vi "Compute DistanceTo AprilTag Ver 2.vi"(8 "Height to center of target from floor (hp (in))":dbl=10.875 format="%#_13g", 9 "Screen resolution pixels Height (Ry)":dbl=600.0 format="%#_13g", 10 "Target Vertical pixels bottom - top (pixels)":dbl=-46.076202392578125 format="%#_13g", 11 "Robot Calibration Cluster":T1={"Camera Height on robot (in)"=6.0, "Camera Angle on the robot (deg)"=5.0, "Camera FOV Vert View Angle (deg)"=1.0, "Camera FOV Hor View Angle (deg)"=26.5, "Camera Focal Length (mm)"=10.0, "Target size (in)"=6.5, "Distance Correction Factor"=3.952} {"Distance Correction Factor" format="%#_13g"; "Camera FOV Hor View Angle (deg)" format="%#_13g"; "Camera Focal Length (mm)" format="%#_13g"; "Target size (in)" format="%#_13g"; "Camera FOV Vert View Angle (deg)" format="%#_13g"; "Camera Angle on the robot (deg)" format="%#_13g"; "Camera Height on robot (in)" format="%#_13g"}) -> (2 "Distance from camera to apriltag center (in)":dbl format="%.2f")   [LabVIEW 2025]
uses:
  Camera Info.ctl
panel:
  out "Straight Line DIstance (in)":dbl
  # "These Items are inputs"
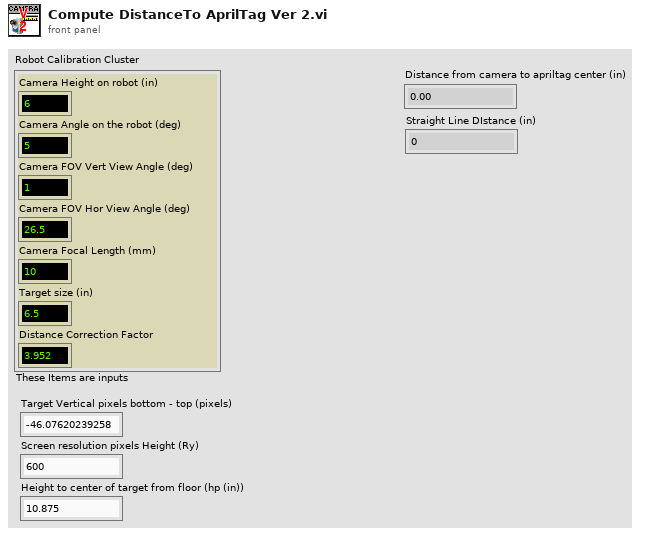
[diagram p1: front panel]
types:
  T1 = typedef "Camera Info.ctl" = cluster{"Camera Height on robot (in)":dbl, "Camera Angle on the robot (deg)":dbl, "Camera FOV Vert View Angle (deg)":dbl, "Camera FOV Hor View Angle (deg)":dbl, "Camera Focal Length (mm)":dbl, "Target size (in)":dbl, "Distance Correction Factor":dbl}
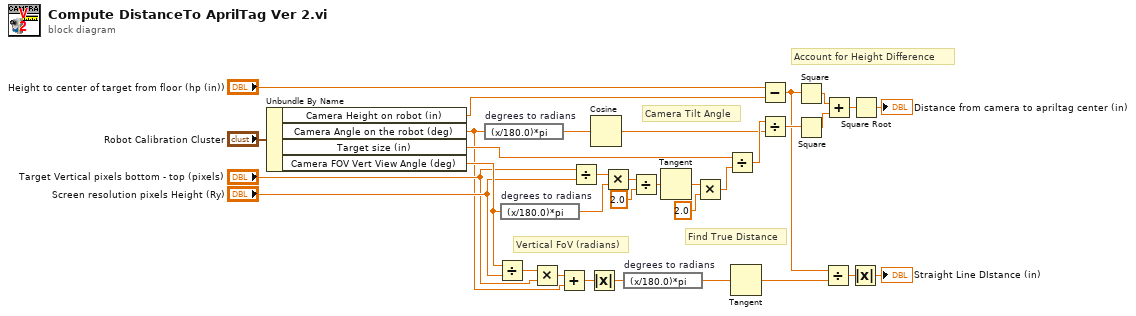
[diagram p0: block diagram]
diagram:
  # "Camera Tilt Angle"
  # "Account for Height Difference"
  # "Find True Distance"
  # "Vertical FoV (radians)"
  n1 = Unbundle By Name("Robot Calibration Cluster") -> ("Camera Height on robot (in)"=w3:dbl, "Camera Angle on the robot (deg)"=w11:dbl, "Target size (in)"=w19:dbl, "Camera FOV Vert View Angle (deg)"=w16:dbl)
  n2 = expression code="(x/180.0)*pi" "degrees to radians"(w11) -> (w17:dbl)
  n3 = Divide(x=w16, y="Screen resolution pixels Height (Ry)") -> (x/y=w14:dbl)
  n4 = expression code="(x/180.0)*pi" "degrees to radians"(w16) -> (w28:dbl)
  n5 = Multiply(x=w14, y="Target Vertical pixels bottom - top (pixels)") -> (x*y=w12:dbl)
  n6 = Add(x=w12, y=w11) -> (x+y=w10:dbl)
  n7 = Divide(x="Target Vertical pixels bottom - top (pixels)", y="Screen resolution pixels Height (Ry)") -> (x/y=w29:dbl)
  n8 = Absolute Value(x=w10) -> (abs(x)=w9:dbl)
  n9 = Cosine(x=w17) -> (cos(x)=w22:dbl)
  n10 = Multiply(x=w29, y=w28) -> (x*y=w27:dbl)
  n11 = expression code="(x/180.0)*pi" "degrees to radians"(w9) -> (w8:dbl)
  n12 = Divide(x=w27, y=2.0) -> (x/y=w25:dbl)
  n13 = Tangent(1:w25) -> (0:w24:dbl)
  n14 = Multiply(x=w24, y=2.0) -> (x*y=w32:dbl)
  n15 = Divide(x=w19, y=w32) -> (x/y=w23:dbl)
  n16 = Tangent(1:w8) -> (0:w7:dbl)
  n17 = Subtract(x="Height to center of target from floor (hp (in))", y=w3) -> (x-y=w20:dbl)
  n18 = Divide(x=w23, y=w22) -> (x/y=w21:dbl)
  n19 = Square(x=w20) -> (x^2=w4:dbl)
  n20 = Square(x=w21) -> (x^2=w5:dbl)
  n21 = Divide(x=w20, y=w7) -> (x/y=w6:dbl)
  n22 = Add(x=w4, y=w5) -> (x+y=w30:dbl)
  n23 = Absolute Value(x=w6) -> (abs(x)=→"Straight Line DIstance (in)":dbl)
  n24 = Square Root(x=w30) -> (sqrt(x)=→"Distance from camera to apriltag center (in)":dbl)
